vi "epx_Update Vector Properties.vi"(8 "error in (no error)":errorcluster, 9 "Display State In":T2={"BGColor"=0, "FGColor"=0, "GridColor"=9868950, "Number of Polar Grids"=12, "Number of Circle Grids"=4, "Vector.Active"=0, "Vectors.Properties"=[], "Height"=0, "Width"=0} {"Number of Circle Grids" min=1 max=100 step=1; "Number of Polar Grids" min=1 max=100 step=1}, 10 "Data In":T1, 11 "Vector Diagram":refnum<vi>) -> (0 "error out":errorcluster, 3 "Vector Diagram out":refnum<vi>)   [LabVIEW 2011, in "NI_EP_Basic.lvlib" / "EPX Vector Diagram.xctl"]
uses:
  <vilib>/addons/Electrical Power/Basic/Controls/Vector Diagram/EPX Vector Diagram.xctl
  <vilib>/addons/Electrical Power/Basic/Controls/Vector Diagram/Abilities/epx_Vector Diagram State.ctl
  <vilib>/addons/Electrical Power/Basic/Controls/Vector Diagram/SubVIs/epx_Vector Type.ctl
  <vilib>/addons/Electrical Power/Basic/Controls/Vector Diagram/Abilities/epx_Vector Diagram Data.ctl
  <vilib>/addons/Electrical Power/Basic/NI_EP_Basic.lvlib
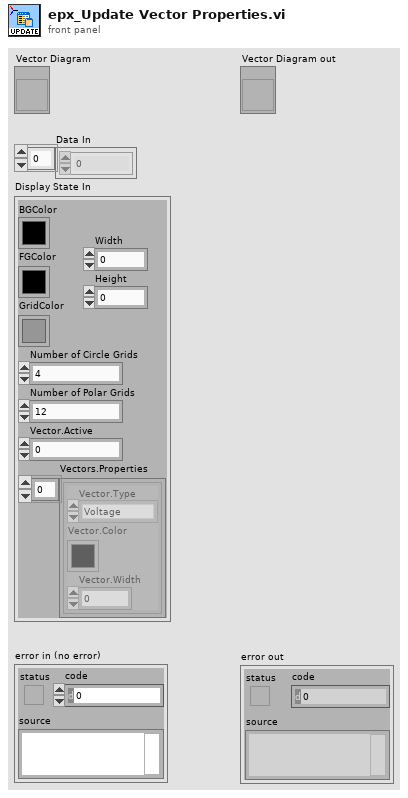
[diagram p1: front panel]
types:
  T1 = typedef "NI_EP_Basic.lvlib/EPX Vector Diagram.xctl/epx_Vector Diagram Data.ctl" = cdb[]
  T2 = typedef "NI_EP_Basic.lvlib/EPX Vector Diagram.xctl/epx_Vector Diagram State.ctl" = cluster{"BGColor":u32, "FGColor":u32, "GridColor":u32, "Number of Polar Grids":i32, "Number of Circle Grids":i32, "Vector.Active":i32, "Vectors.Properties":cluster{"Vector.Type":T3, "Vector.Color":u32, "Vector.Width":u8}[], "Height":u32, "Width":u32}
  T3 = typedef "NI_EP_Basic.lvlib/epx_Vector Type.ctl" = enum16{"Voltage", "Current"}
  T4 = cluster{"BGColor":bool, "FGColor":bool, "GridColor":bool, "Number of Polar Grids":bool, "Number of Circle Grids":bool, "Vector.Active":bool, "Vectors.Properties":cluster{"Vector.Type":bool, "Vector.Color":bool, "Vector.Width":bool}[], "Height":bool, "Width":bool}
  T5 = cluster{"Vector.Type":bool, "Vector.Color":bool, "Vector.Width":bool}[]
  T6 = cluster{"Vector.Type":T3, "Vector.Color":u32, "Vector.Width":u8}[]
  T7 = cluster{"Vector.Type":T3, "Vector.Color":u32, "Vector.Width":u8}
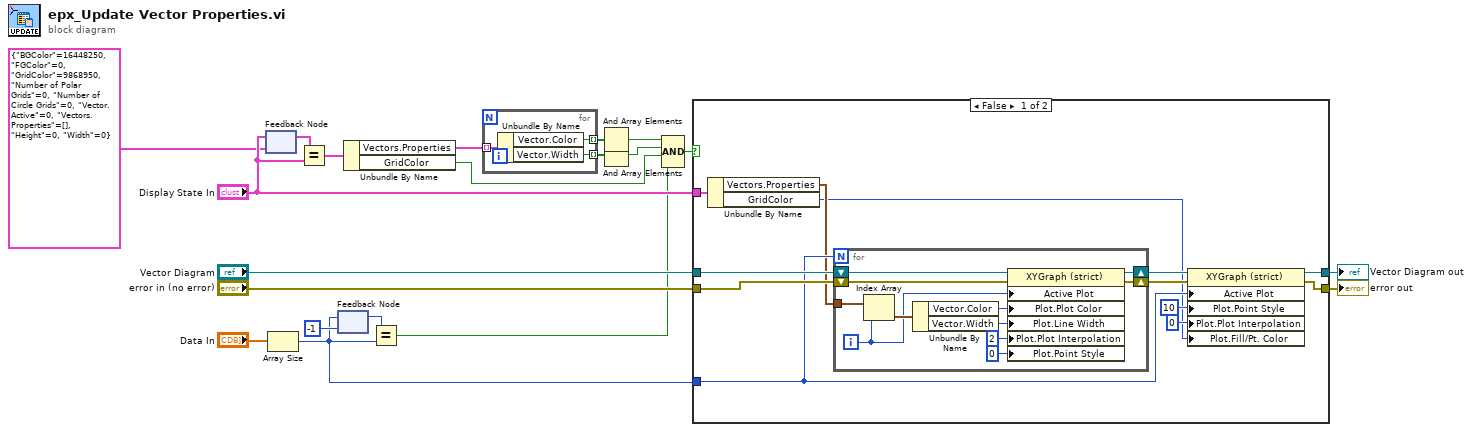
[diagram p0: block diagram]
diagram:
  n1 = feedback-in #1("Display State In") -> ()
  n2 = feedback #1(T2 {"BGColor"=16448250, "FGColor"=0, "GridColor"=9868950, "Number of Polar Grids"=0, "Number of Circle Grids"=0, "Vector.Active"=0, "Vectors.Properties"=[], "Height"=0, "Width"=0} ("Display State In")) -> (w15:T2)
  n3 = Array Size(array="Data In") -> (size(s)=w3:i32)
  n4 = Equal?(x=w15, y="Display State In") -> (x = y?=w13:T4)
  n5 = feedback-in #2(w3) -> ()
  n6 = feedback #2(-1) -> (w16:i32)
  n7 = Unbundle By Name(w13) -> ("Vectors.Properties"=w12:T5, "GridColor"=w2:bool)
  n8 = Equal?(x=w16, y=w3) -> (x = y?=w1:bool)
  n9 = for {
    tunnel: w12 -> [w23] mode=indexing
    tunnel: [w22] -> w11 mode=indexing
    tunnel: [w21] -> w7 mode=indexing
    n10 = Unbundle By Name(w23) -> ("Vector.Color"=w22:bool, "Vector.Width"=w21:bool)
  }
  n11 = And Array Elements(Boolean array=w11) -> (logical AND=w10:bool)
  n12 = And Array Elements(Boolean array=w7) -> (logical AND=w6:bool)
  n13 = Compound Arithmetic op=AND(w10, w6, w2, w1) -> (w9:bool)
  n14 = case shown="False" w9 {
    tunnel: [w30 w47] -> w20
    tunnel: [w31 w48] -> w19
    tunnel: "Vector Diagram" -> [w29 w48]
    tunnel: "error in (no error)" -> [w28 w47]
    tunnel: "Display State In" -> [w27 _]
    tunnel: w3 -> [w26 _]
    frame False {
      n15 = Unbundle By Name(w27) -> ("Vectors.Properties"=w25:T6, "GridColor"=w24:u32)
      n16 = for {
        N: w26 -> [_]
        tunnel: w25 -> [w38]
        shift-right: [w43] -> w34
        shift-left: w28 -> [w42]
        shift-right: [w41] -> w35
        shift-left: w29 -> [w44]
        i -> [w36]
        n17 = Index Array(array=w38, index=w36) -> (element=w37:T7)
        n18 = Unbundle By Name(w37) -> ("Vector.Color"=w46:u32, "Vector.Width"=w45:u8)
        n19 = property on="Property Node" class="XYGraph (strict)"(reference=w44, error in=w42, "Active Plot"=w36, "Plot.Plot Color"=w46, "Plot.Line Width"=w45, "Plot.Plot Interpolation"=u8 2, "Plot.Point Style"=u8 0) -> (reference out=w41:refnum<vi>, error out=w43:errorcluster)
      }
      n20 = property on="Property Node" class="XYGraph (strict)"(reference=w35, error in=w34, "Active Plot"=w26, "Plot.Point Style"=u8 10 ("Plot.Plot Interpolation"), "Plot.Plot Interpolation"=u8 0 ("Plot.Point Style"), "Plot.Fill/Pt. Color"=w24) -> (reference out=w31:refnum<vi>, error out=w30:errorcluster)
    }
    frame True {
    }
  }
  "error out" <- w20
  "Vector Diagram out" <- w19
